vi "TestWriteMultipleImages.vi"() -> ()   [LabVIEW 2012]
uses:
  LVTiffWriter.lvlib
panel:
  in  "Compress?":bool=TRUE
  out "Image":T1(plugin-control)
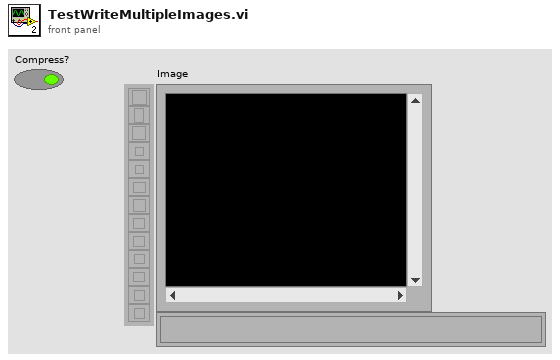
[diagram p1: front panel]
types:
  T1 = typedef "IMAQ Image.ctl" = refnum<image>
  T2 = typedef "Image Type" = u32
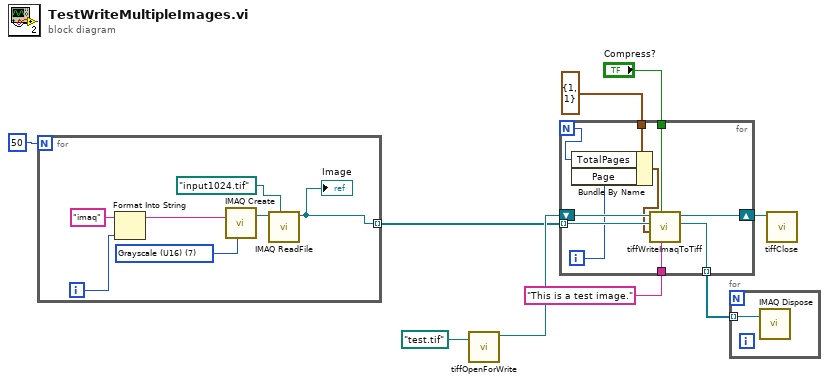
[diagram p0: block diagram]
diagram:
  n1 = for {
    N: 50 -> [_]
    tunnel: [w13] -> w5 mode=indexing
    i -> [w11]
    w14 = T2 7 items=["Grayscale (U8)", "Grayscale (I16)", "Grayscale (SGL)", "Complex (CSG)", "RGB (U32)", "HSL (U32)", "RGB (U64)", "Grayscale (U16)"] ("Image Type")
    n2 = Format Into String(initial string="imaq", w11) -> (resulting string=w12:string)  [unwired: 2 in, 1 out]
    n3 = call "IMAQ Create"("Image Name"=w12, "Image Type"=w14) -> ("New Image"=w15:T1)  [unwired: 3 in, 1 out]
    n4 = call "IMAQ ReadFile"("File Path"=path "input1024.tif", "Image"=w15) -> ("Image Out"=w13:T1)  [unwired: 5 in, 4 out]
    "Image" <- w13
  }
  n5 = call "tiffOpenForWrite.vi"("Path"=path "test.tif") -> ("TiffOut"=w6:refnum<k24>)  [unwired: 10 in]
  n6 = for {
    N -> [w21]
    tunnel: "Compress?" -> [w25]
    tunnel: w5 -> [w23] mode=indexing
    shift-right: [w26] -> w9
    shift-left: w6 -> [w24]
    tunnel: cluster{"Page":i32, "TotalPages":i32} {"Page"=1, "TotalPages"=1} ("Multipage") -> [w22]
    tunnel: [w18] -> w2 mode=indexing
    tunnel: "This is a test image." ("ImageDescription") -> [w17]
    i -> [w20]
    n7 = Bundle By Name(cluster=w22, "TotalPages"=w21, "Page"=w20) -> (w19:cluster{"Page":i32, "TotalPages":i32})
    n8 = call "tiffWriteImaqToTiff.vi"("ImageDescription"=w17, "Compress?"=w25, "Multipage"=w19, "ImaqIn"=w23, "TiffIn"=w24) -> ("ImaqOut"=w18:T1, "TiffOut"=w26:refnum<k24>)  [unwired: 5 in]
  }
  n9 = for {
    tunnel: w2 -> [w27] mode=indexing
    n10 = call "IMAQ Dispose"("Image"=w27) -> ()  [unwired: 5 in, 1 out]
  }
  n11 = call "tiffClose.vi"("Tiff in"=w9) -> ()  [unwired: 10 in, 1 out]
